vi "AudioTest.Normalize DB Plot.vi"(10 "Avg DB":dbl, 11 "Plot DB":cluster{"F":dbl[], "M":dbl[]}={"F"=[19993.502974545063, 19129.054798935926, 18296.045129605558, 17499.306408924178, 16737.263341271664, 16008.405001718565, 15311.286290675285, 14644.525026116988, 14006.799225066536, 13396.844519115479, 12813.451535229751, 12255.463573373227, 11721.77438607659, 11211.325744569638, 10723.105634000056, 10256.146092611636, 9809.5212292847, 9382.345570839127, 8973.772149157394, 8582.990891663025, 8209.227002426016, 7851.739433110429, 7509.819389158058, 7182.788946270568, 6869.999716958011, 6570.831533763757, 6284.691240202259, 6011.011513283507, 5749.249726048645, 5498.886891378922, 5259.426617984524, 5030.394134568383, 4811.335337232323, 4601.815902710357, 4401.420420464474, 4209.7515697419885, 4026.4293305773585, 3851.0902332129604, 3683.386635342684, 3522.986033342509, 3369.5704036968623, 3222.8355713080086, 3082.49060711571, 2948.257251457507, 2819.869361635349, 2697.0723849711394, 2579.622853659401, 2467.2879023025293, 2359.8448062202124, 2257.0805393732953, 2158.7913526287102, 2064.7823694039566, 1974.8671996182454, 1888.8675697522515, 1806.6129695670577, 1727.940314125843, 1652.6936203253547, 1580.7236976517197, 1511.8878523786307, 1446.0496047503643, 1383.0784182181944, 1322.8494407451155, 1265.2432572441312, 1210.1456527777157, 1157.4473861455042, 1107.0439732729624, 1058.8354800696895, 1012.7263242673238, 968.6250859261445, 926.4443261775026, 886.1004138471127, 847.5133596647895, 810.6066576615648, 775.3071334308887, 741.5447991661738, 709.2527147742612, 678.3668552594401, 648.8259835656797, 620.5715295660932, 593.5474735329731, 567.7002352708697, 542.9785678445741, 519.3334559706822, 496.71801883655576, 475.0874171503279, 454.39876423914063, 434.6110410174567, 415.685014671574, 397.58316085539934, 380.26958920615516, 363.70997247075184, 347.87147810282926, 332.72270335444307, 318.23361300055757, 304.37547966651175, 291.1208271022314, 278.44337547002476, 266.3179894009186, 254.72062807932286, 243.62829752569326, 233.01900520012987, 222.8717162178992, 213.16631165906742, 203.88354878707116, 195.00502283537796, 186.51313041650593, 178.3910348020954, 170.622632474182, 163.19252109791395, 156.08596911525854, 149.2888864597299, 142.78779668446768, 136.56981013311903, 130.62259852965386, 124.93437041460261, 119.49384783050523, 114.29024391334877, 109.31324156999352, 104.55297296991515, 0.0], "M"=[-85.9370770167748, -99.778395504104, -83.11095984415557, -81.77543077538515, -90.27946954622428, -84.93782886679098, -76.63235717176379, -94.41593737291855, -81.09487652347323, -79.73031438457498, -80.33524317211999, -83.09734063798807, -84.30813915558306, -85.25107725367418, -81.56613893474338, -79.73906325412882, -85.15117761670643, -84.84990171730556, -77.672887972436, -89.53752158355618, -85.33337554491749, -90.4373862783058, -80.5030809948349, -84.75064105050096, -80.69841153333357, -92.4921725301016, -81.6538418757633, -82.85905182376924, -79.21423206592686, -81.6387059073133, -81.11646687271508, -83.04152622868713, -88.33602202912445, -83.38154714004519, -88.72775750258933, -80.98443084351632, -73.05532734948075, -70.1551554704772, -71.035137141613, -64.02038640229722, -74.0926125747394, -63.70041248227204, -61.44225905249079, -65.012671399401, -62.22258698666924, -68.11415583475622, -60.2691998871055, -58.27708426816994, -51.374042698447504, -44.672298612394, -46.35566537856021, -45.02841502570413, -52.48018936603423, -53.87580558626168, -49.96698952505654, -44.19340441383534, -43.4027934169752, -37.684193953897804, -36.05360358765683, -41.93669602167696, -44.144181336907955, -46.76643640988917, -39.267847996982404, -37.695992175046385, -46.034400474420984, -48.637036012377266, -46.389140343304824, -38.17294392250851, -42.689223937286584, -43.657480149200595, -51.74372728079939, -35.84983709618854, -39.238287399407106, -36.78388253903451, -58.277560826454, -27.422227890722652, -36.495096712247566, -54.257716007328156, -42.768442512703714, -49.3290323125036, -62.76898977413002, -37.96268155745586, -34.625054525971, -37.008530356666604, -32.4242252469013, -39.35992488588547, -40.28752804562661, -38.75156186672819, -34.36299303601085, -33.36901366976663, -33.34686403991625, -40.33693625797695, -38.91025090748522, -36.37908780803699, -39.07781448777433, -43.92731237758593, -37.510661082962095, -38.293806773881386, -35.24021826259905, -34.159341786903, -33.48669692941214, -41.40004423486004, -35.80458501672772, -35.396080829708666, -33.27215417774858, -32.72827949088403, -30.51433428135859, -36.02637989722959, -42.728555561627545, -42.38800729126141, -53.95638380582021, -70.74014358132499, -72.40034495946185, -46.0259591055895, -41.05349184528848, -46.582707455893065, -67.75623188725073, -64.14424048230943, -73.57528464520568, 0.0]}) -> (3 "Norm Plot":cluster{"F":dbl[], "M":dbl[]}={"F"=[19993.502974545063, 19129.054798935926, 18296.045129605558, 17499.306408924178, 16737.263341271664, 16008.405001718565, 15311.286290675285, 14644.525026116988, 14006.799225066536, 13396.844519115479, 12813.451535229751, 12255.463573373227, 11721.77438607659, 11211.325744569638, 10723.105634000056, 10256.146092611636, 9809.5212292847, 9382.345570839127, 8973.772149157394, 8582.990891663025, 8209.227002426016, 7851.739433110429, 7509.819389158058, 7182.788946270568, 6869.999716958011, 6570.831533763757, 6284.691240202259, 6011.011513283507, 5749.249726048645, 5498.886891378922, 5259.426617984524, 5030.394134568383, 4811.335337232323, 4601.815902710357, 4401.420420464474, 4209.7515697419885, 4026.4293305773585, 3851.0902332129604, 3683.386635342684, 3522.986033342509, 3369.5704036968623, 3222.8355713080086, 3082.49060711571, 2948.257251457507, 2819.869361635349, 2697.0723849711394, 2579.622853659401, 2467.2879023025293, 2359.8448062202124, 2257.0805393732953, 2158.7913526287102, 2064.7823694039566, 1974.8671996182454, 1888.8675697522515, 1806.6129695670577, 1727.940314125843, 1652.6936203253547, 1580.7236976517197, 1511.8878523786307, 1446.0496047503643, 1383.0784182181944, 1322.8494407451155, 1265.2432572441312, 1210.1456527777157, 1157.4473861455042, 1107.0439732729624, 1058.8354800696895, 1012.7263242673238, 968.6250859261445, 926.4443261775026, 886.1004138471127, 847.5133596647895, 810.6066576615648, 775.3071334308887, 741.5447991661738, 709.2527147742612, 678.3668552594401, 648.8259835656797, 620.5715295660932, 593.5474735329731, 567.7002352708697, 542.9785678445741, 519.3334559706822, 496.71801883655576, 475.0874171503279, 454.39876423914063, 434.6110410174567, 415.685014671574, 397.58316085539934, 380.26958920615516, 363.70997247075184, 347.87147810282926, 332.72270335444307, 318.23361300055757, 304.37547966651175, 291.1208271022314, 278.44337547002476, 266.3179894009186, 254.72062807932286, 243.62829752569326, 233.01900520012987, 222.8717162178992, 213.16631165906742, 203.88354878707116, 195.00502283537796, 186.51313041650593, 178.3910348020954, 170.622632474182, 163.19252109791395, 156.08596911525854, 149.2888864597299, 142.78779668446768, 136.56981013311903, 130.62259852965386, 124.93437041460261, 119.49384783050523, 114.29024391334877, 109.31324156999352, 104.55297296991515, 0.0], "M"=[-85.9370770167748, -99.778395504104, -83.11095984415557, -81.77543077538515, -90.27946954622428, -84.93782886679098, -76.63235717176379, -94.41593737291855, -81.09487652347323, -79.73031438457498, -80.33524317211999, -83.09734063798807, -84.30813915558306, -85.25107725367418, -81.56613893474338, -79.73906325412882, -85.15117761670643, -84.84990171730556, -77.672887972436, -89.53752158355618, -85.33337554491749, -90.4373862783058, -80.5030809948349, -84.75064105050096, -80.69841153333357, -92.4921725301016, -81.6538418757633, -82.85905182376924, -79.21423206592686, -81.6387059073133, -81.11646687271508, -83.04152622868713, -88.33602202912445, -83.38154714004519, -88.72775750258933, -80.98443084351632, -73.05532734948075, -70.1551554704772, -71.035137141613, -64.02038640229722, -74.0926125747394, -63.70041248227204, -61.44225905249079, -65.012671399401, -62.22258698666924, -68.11415583475622, -60.2691998871055, -58.27708426816994, -51.374042698447504, -44.672298612394, -46.35566537856021, -45.02841502570413, -52.48018936603423, -53.87580558626168, -49.96698952505654, -44.19340441383534, -43.4027934169752, -37.684193953897804, -36.05360358765683, -41.93669602167696, -44.144181336907955, -46.76643640988917, -39.267847996982404, -37.695992175046385, -46.034400474420984, -48.637036012377266, -46.389140343304824, -38.17294392250851, -42.689223937286584, -43.657480149200595, -51.74372728079939, -35.84983709618854, -39.238287399407106, -36.78388253903451, -58.277560826454, -27.422227890722652, -36.495096712247566, -54.257716007328156, -42.768442512703714, -49.3290323125036, -62.76898977413002, -37.96268155745586, -34.625054525971, -37.008530356666604, -32.4242252469013, -39.35992488588547, -40.28752804562661, -38.75156186672819, -34.36299303601085, -33.36901366976663, -33.34686403991625, -40.33693625797695, -38.91025090748522, -36.37908780803699, -39.07781448777433, -43.92731237758593, -37.510661082962095, -38.293806773881386, -35.24021826259905, -34.159341786903, -33.48669692941214, -41.40004423486004, -35.80458501672772, -35.396080829708666, -33.27215417774858, -32.72827949088403, -30.51433428135859, -36.02637989722959, -42.728555561627545, -42.38800729126141, -53.95638380582021, -70.74014358132499, -72.40034495946185, -46.0259591055895, -41.05349184528848, -46.582707455893065, -67.75623188725073, -64.14424048230943, -73.57528464520568, 0.0]})   [LabVIEW 2018]
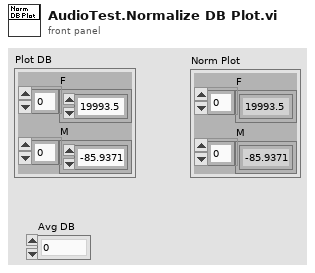
[diagram p1: front panel]
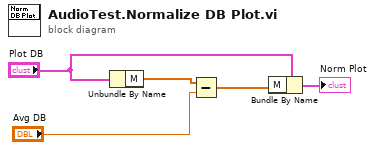
[diagram p0: block diagram]
diagram:
  n1 = Unbundle By Name("Plot DB") -> ("M"=w5:dbl[])
  n2 = Subtract(x=w5, y="Avg DB") -> (x-y=w2:dbl[])
  n3 = Bundle By Name(cluster="Plot DB", "M"=w2) -> (→"Norm Plot":cluster{"F":dbl[], "M":dbl[]})
